vi "lab_3_lab.vi"() -> ()   [LabVIEW 2016]
panel:
  in  "Exit":bool
  in  "stop":bool
  out "time":dbl
  out "Waveform Graph":dynamicdata(graph)
  out "Waveform Chart":dynamicdata(graph)
  in  "Freq":dbl(knob) scale=0.0..10.0
  in  "Amplitude":dbl(knob) scale=0.0..10.0
  in  "Offset":dbl(knob) scale=0.0..10.0
  in  "Select signal":i16(knob) scale=0.0..2.0
  in  "Start":bool
  out "raw data file":refnum<file>
  out "Folder_Name":string
  in  "DATE":string
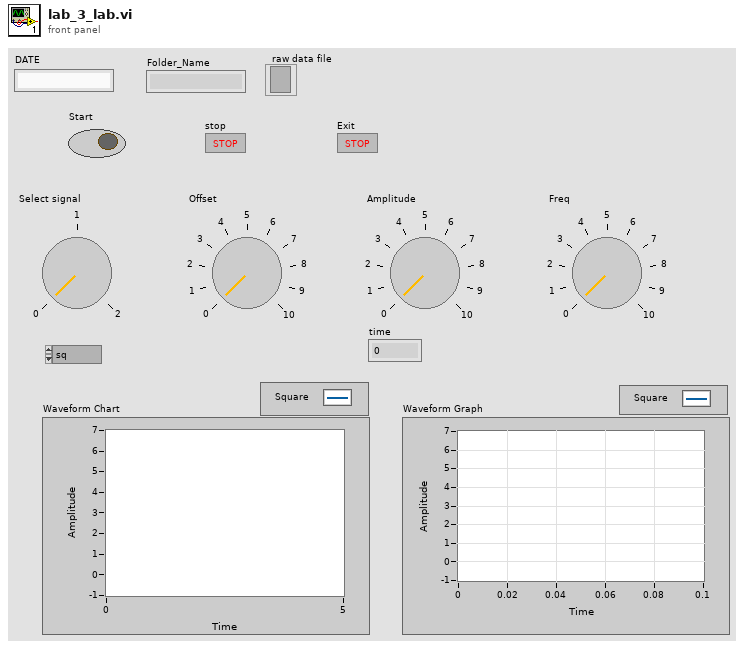
[diagram p1: front panel]
types:
  T1 = enum16{"open", "replace", "create", "open or create", "replace or create", "replace or create with confirmation"}
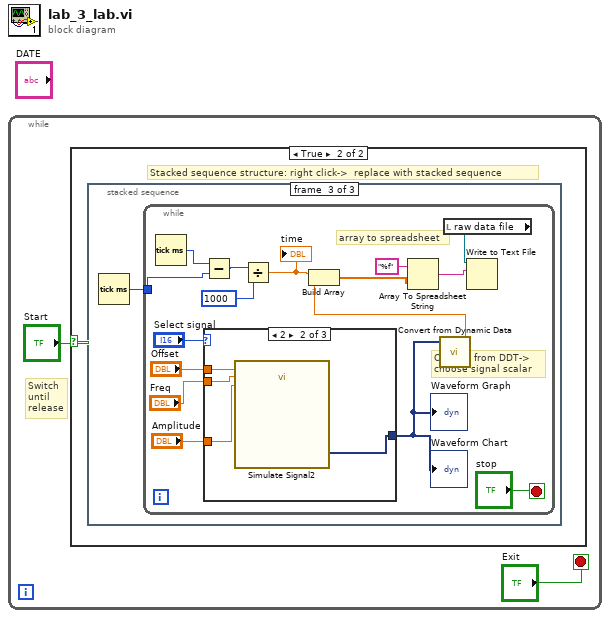
[diagram p0: block diagram]
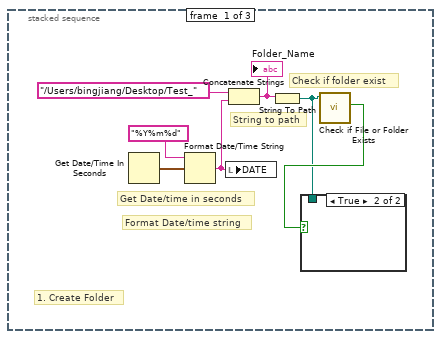
[diagram p3: hidden frame]
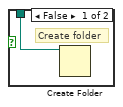
[diagram p4: hidden frame]
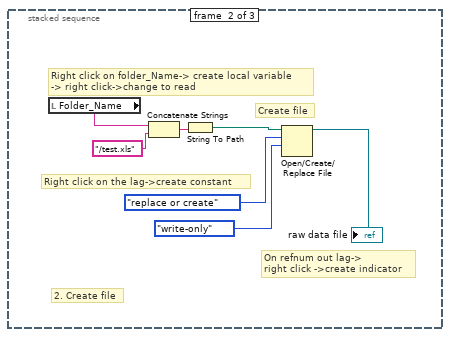
[diagram p5: hidden frame]
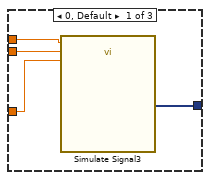
[diagram p6: hidden frame]
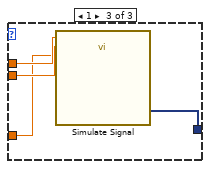
[diagram p7: hidden frame]
diagram:
  n1 = while {
    stop <- "Exit" stop-if-true
    # "Switch\nuntil\nrelease"
    n2 = case shown="True" "Start" {
      frame False {
      }
      frame True {
        # "Stacked sequence structure: right click->  replace with stacked sequence"
        n3 = stacked-sequence {
          frame #0 {
            # "1. Create Folder"
            # "Check if folder exist"
            # "String to path"
            # "Get Date/time in seconds"
            # "Format Date/time string"
            n4 = Get Date/Time In Seconds() -> (seconds since 1Jan1904=w9:timestamp)
            n5 = Format Date/Time String(time format string (%c)="%Y%m%d", seconds (now)=w9) -> (date/time string=w7:string)  [unwired: 1 in]
            n6 = local write "DATE"(w7) -> ()
            n7 = Concatenate Strings("/Users/bingjiang/Desktop/Test_" ("string"), w7) -> (w5:string)
            "Folder_Name" <- w5
            n8 = String To Path(string=w5) -> (path=w3:path)
            n9 = call <vilib>:"Check if File or Folder Exists.vi"("path"=w3) -> ("file or folder exists?"=w4:bool)  [unwired: 8 in, 2 out]
            n10 = case shown="True" w4 {
              tunnel: w3 -> [w10 _]
              frame False {
                # "Create folder"
                n11 = Create Folder(path (use dialog)=w10) -> ()  [unwired: 2 in, 3 out]
              }
              frame True {
              }
            }
          }
          frame #1 {
            # "2. Create file"
            # "On refnum out lag->\nright click ->create indicator"
            # "Right click on the lag->create constant"
            # "Create file"
            # "Right click on folder_Name-> create local variable\n-> right click->change to read"
            n12 = local read "Folder_Name"() -> (w17:string)
            n13 = Concatenate Strings(w17, "/test.xls") -> (w15:string)
            n14 = String To Path(string=w15) -> (path=w14:path)
            n15 = Open/Create/Replace File(file path (use dialog)=w14, operation (0:open)=T1."replace or create", access (0:read/write)=enum16{"read/write", "read-only", "write-only"}."write-only") -> (refnum out=→"raw data file":refnum<file>)  [unwired: 3 in, 2 out]
          }
          frame #2 {
            n16 = Tick Count (ms)() -> (millisecond timer value=w18:u32)
            n17 = while {
              tunnel: w18 -> [w20]
              stop <- "stop" stop-if-true
              # "Convert from DDT->\nchoose signal scalar"
              # "array to spreadsheet"
              n18 = Tick Count (ms)() -> (millisecond timer value=w26:u32)
              n19 = Subtract(x=w26, y=w20) -> (x-y=w25:u32)
              n20 = case shown="2" "Select signal" {
                tunnel: "Offset" -> [w38 w41 w46]
                tunnel: "Freq" -> [w37 w40 w45]
                tunnel: "Amplitude" -> [w36 w39 w44]
                tunnel: [w35 w42 w43] -> w27
                frame 0, Default {
                  n21 = call "Simulate Signal3"("Offset"=w38, "Frequency"=w37, "Amplitude"=w36) -> ("Square"=w35:dynamicdata)  [unwired: 11 in, 1 out]
                }
                frame 2 {
                  n22 = call "Simulate Signal2"("Offset"=w41, "Frequency"=w40, "Amplitude"=w39) -> ("Triangle"=w42:dynamicdata)  [unwired: 11 in, 1 out]
                }
                frame 1 {
                  n23 = call "Simulate Signal"("Offset"=w46, "Frequency"=w45, "Amplitude"=w44) -> ("Sine"=w43:dynamicdata)  [unwired: 11 in, 1 out]
                }
              }
              "Waveform Graph" <- w27
              "Waveform Chart" <- w27
              n24 = Divide(x=w25, y=u32 1000) -> (x/y=w23:dbl)
              "time" <- w23
              n25 = call "Convert from Dynamic Data"("Dynamic Data Type"=w27) -> ("Scalar"=w21:dbl)  [unwired: 3 in]
              n26 = Build Array(w23, w21) -> (w22:dbl[])
              n27 = Array To Spreadsheet String(array=w22, 3:"%f" ("format string")) -> (spreadsheet string=w34:string)  [unwired: 1 in]
              n28 = local read "raw data file"() -> (w32:refnum<file>)
              n29 = Write to Text File(file (use dialog)=w32, text=w34) -> ()  [unwired: 2 in, 3 out]
            }
          }
        }
      }
    }
  }
